vi "Three_Tote_works_3_21.vi"(11 "3_Tote_Enable":bool=TRUE) -> ()   [LabVIEW 2014]
uses:
  General_VI/Global Var.vi
panel:
  in  "Time _To_Drive_1_Tote":i32=8000
  in  "Extend_Flipper_Time":i32=500
  in  "Open_Infeed_time":i32=800
  # "Static Tunning Values"
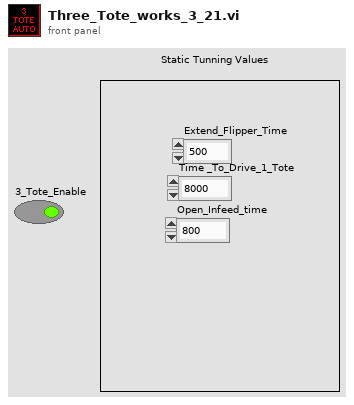
[diagram p1: front panel]
types:
  T1 = cluster{"Open_Infeed_time":i32, "Extend_Flipper_Time":i32, "Time _To_Drive_1_Tote":i32}
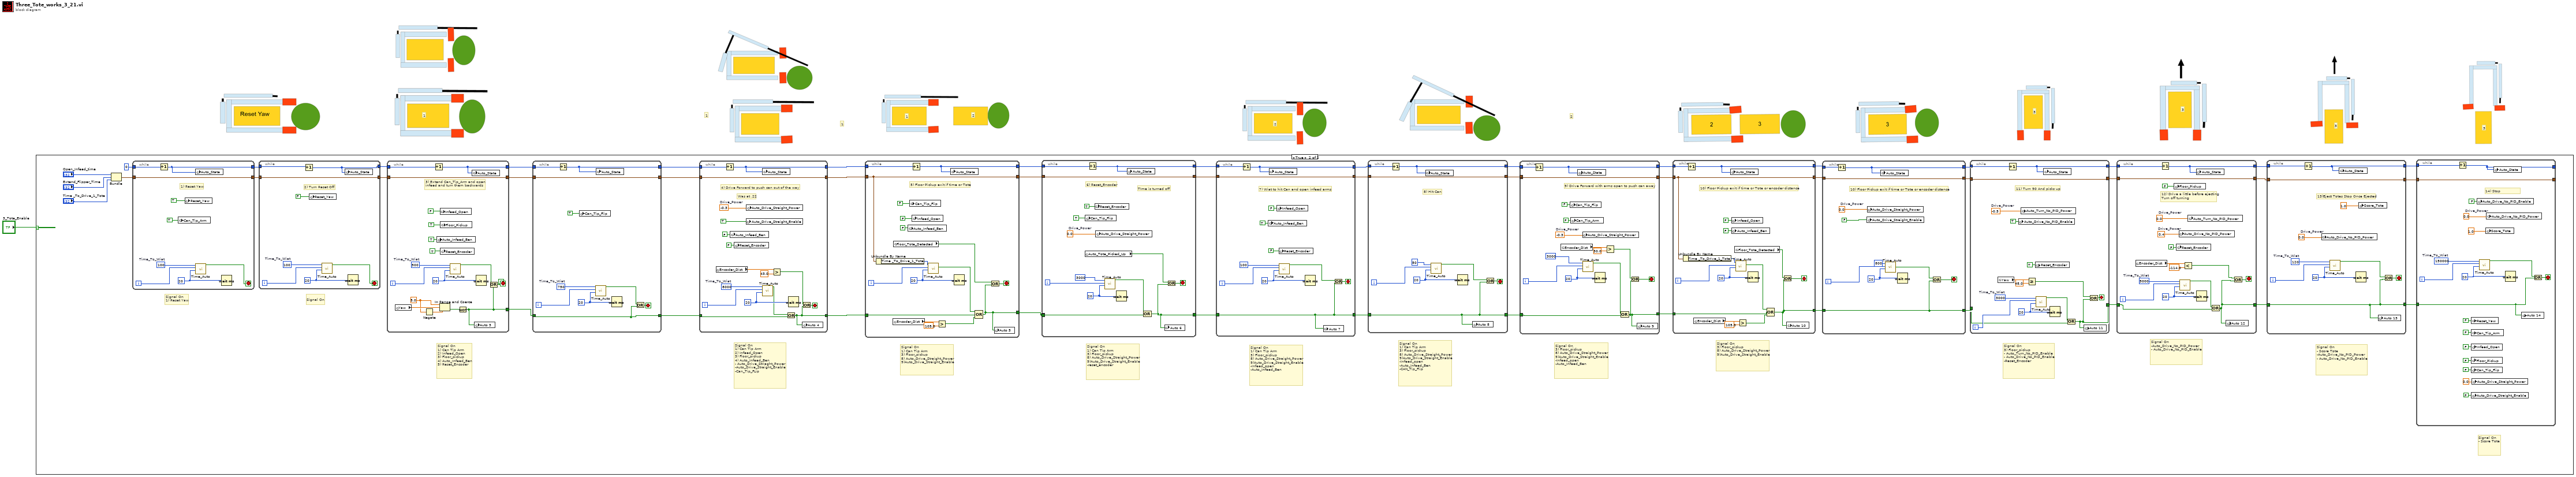
[diagram p0: block diagram]
diagram:
  # "3"
  # "3"
  # "3"
  # "3"
  # "2"
  # "2"
  # "2"
  # "1"
  # "1"
  # "1"
  # "1"
  n1 = case shown="True" "3_Tote_Enable" {
    frame False {
    }
    frame True {
      # "Signal On\n1) Can Tip Arm\n2) Infeed_Open\n3) Floor_pickup\n4) Auto_Infeed_Ben\n- Auto_Drive_Striaght_Power\n-Auto_Drive_Straight_Enable\n-Can_Tip_FLip"
      # "Signal On\n- Score Tote"
      # "Signal On\n- Score Tote\n-Auto_Drive_No_PID_Power\n- Auto_Drive_No_PID_Enable"
      # "Signal On\n-Auto_Drive_No_PID_Power\n- Auto_Drive_No_PID_Enable"
      # "Signal On\n3) Floor_pickup\n- Auto_Turn_No_PID_Enable\n- Auto_Drive_No_PID_Enable\n-Reset_Encoder"
      # "Signal On\n3) Floor_pickup\n8) Auto_Drive_Straight_Power\n9)Auto_Drive_Straight_Enable"
      # "Signal On\n3) Floor_pickup\n8) Auto_Drive_Straight_Power\n9)Auto_Drive_Straight_Enable\n-Infeed_open\n-Auto_Infeed_Ben"
      # "Signal On\n1) Can Tip Arm\n3) Floor_pickup\n8) Auto_Drive_Straight_Power\n9)Auto_Drive_Straight_Enable\n-Infeed_open\n-Auto_Infeed_Ben\n-CAN_Tip_Flip"
      # "Signal On\n1) Can Tip Arm\n3) Floor_pickup\n8) Auto_Drive_Straight_Power\n9)Auto_Drive_Straight_Enable\n-Infeed_open\n-Auto_Infeed_Ben"
      # "Signal On\n1) Can Tip Arm\n3) Floor_pickup\n8) Auto_Drive_Straight_Power\n9)Auto_Drive_Straight_Enable\n-reset_encoder"
      # "Signal On\n1) Can Tip Arm\n3) Floor_pickup\n8) Auto_Drive_Straight_Power\n9)Auto_Drive_Straight_Enable"
      # "Signal On\n1) Can Tip Arm\n2) Infeed_Open\n3) Floor_pickup\n4) Auto_Infeed_Ben\n5) Reset_Encoder"
      # "Signal On"
      # "Signal On\n1) Reset Yaw"
      n2 = Bundle("Open_Infeed_time"="Open_Infeed_time", "Extend_Flipper_Time"="Extend_Flipper_Time", "Time _To_Drive_1_Tote"="Time _To_Drive_1_Tote") -> (w39:T1)  [unwired: 1 in]
      n3 = while {
        tunnel: 0 -> [w262]
        tunnel: [w261] -> w48
        tunnel: w39 -> [w263]
        tunnel: [w263] -> w38
        i -> [w266]
        stop <- w268 stop-if-true
        w267 = u32 20 ("milliseconds to wait")
        w265 = 100  # Time_To_Wiat
        # "1) Reset Yaw"
        n4 = Increment(x=w262) -> (x+1=w261:i32)
        n5 = global write "Global Var.vi" "Can_Tip_Arm"(TRUE) -> ()
        n6 = global write "Global Var.vi" "Reset_Yaw"(TRUE) -> ()
        n7 = global write "Global Var.vi" "Auto_State"(w261) -> ()
        n8 = call "Time_Auto.vi"("Sample_Time"=w267, "Counter"=w266, "Time_to_wait"=w265) -> ("Boolean"=w268:bool)  [unwired: 8 in]
        n9 = Wait (ms)(milliseconds to wait=w267) -> ()  [unwired: 1 out]
      }
      n10 = while {
        tunnel: w48 -> [w253]
        tunnel: [w252] -> w47
        tunnel: w38 -> [w254]
        tunnel: [w254] -> w37
        i -> [w257]
        stop <- w259 stop-if-true
        w258 = u32 20 ("milliseconds to wait")
        w256 = 100  # Time_To_Wiat
        # "2) Turn Reset Off"
        n11 = Increment(x=w253) -> (x+1=w252:i32)
        n12 = global write "Global Var.vi" "Reset_Yaw"(FALSE) -> ()
        n13 = call "Time_Auto.vi"("Sample_Time"=w258, "Counter"=w257, "Time_to_wait"=w256) -> ("Boolean"=w259:bool)  [unwired: 8 in]
        n14 = global write "Global Var.vi" "Auto_State"(w252) -> ()
        n15 = Wait (ms)(milliseconds to wait=w258) -> ()  [unwired: 1 out]
      }
      n16 = while {
        tunnel: w47 -> [w247]
        tunnel: [w246] -> w11
        tunnel: w37 -> [w248]
        tunnel: [w248] -> w12
        tunnel: [w235] -> w14
        i -> [w250]
        stop <- w237 stop-if-true
        w241 = 5.0 ("upper limit")
        w251 = u32 20 ("milliseconds to wait")
        w249 = 500  # Time_To_Wiat
        # "3) Extend Can_Tip_Arm and open \ninfeed and turn them backwards"
        n17 = global read "Global Var.vi" "Yaw"() -> (w243:dbl)
        n18 = Negate(x=w241) -> (-x=w242:dbl)
        n19 = Increment(x=w247) -> (x+1=w246:i32)
        n20 = global write "Global Var.vi" "Auto_Infeed_Ben"(TRUE) -> ()
        n21 = In Range and Coerce(upper limit=w241, x=w243, lower limit=w242) -> (In Range?=w240:bool)  [unwired: 1 out]
        n22 = global write "Global Var.vi" "Infeed_Open"(FALSE) -> ()
        n23 = global write "Global Var.vi" "Floor_Pickup"(TRUE) -> ()
        n24 = global write "Global Var.vi" "Reset_Encoder"(TRUE) -> ()
        n25 = call "Time_Auto.vi"("Sample_Time"=w251, "Counter"=w250, "Time_to_wait"=w249) -> ("Boolean"=w236:bool)  [unwired: 8 in]
        n26 = Not(x=w240) -> (.not. x?=w235:bool)
        n27 = global write "Global Var.vi" "Auto_State"(w246) -> ()
        n28 = global write "Global Var.vi" "Auto 3"(w235) -> ()
        n29 = Wait (ms)(milliseconds to wait=w251) -> ()  [unwired: 1 out]
        n30 = Or(x=w236, y=w235) -> (x .or. y?=w237:bool)
      }
      n31 = while {
        tunnel: w11 -> [w66]
        tunnel: [w65] -> w10
        tunnel: w12 -> [w67]
        tunnel: [w67] -> w9
        tunnel: w14 -> [w61]
        tunnel: [w61] -> w13
        i -> [w69]
        stop <- w64 stop-if-true
        w70 = u32 20 ("milliseconds to wait")
        w68 = 750  # Time_To_Wiat
        n32 = Increment(x=w66) -> (x+1=w65:i32)
        n33 = global write "Global Var.vi" "Can_Tip_Flip"(TRUE) -> ()
        n34 = call "Time_Auto.vi"("Sample_Time"=w70, "Counter"=w69, "Time_to_wait"=w68) -> ("Boolean"=w62:bool)  [unwired: 8 in]
        n35 = global write "Global Var.vi" "Auto_State"(w65) -> ()
        n36 = Wait (ms)(milliseconds to wait=w70) -> ()  [unwired: 1 out]
        n37 = Or(x=w62, y=w61) -> (x .or. y?=w64:bool)
      }
      n38 = while {
        tunnel: w10 -> [w230]
        tunnel: [w229] -> w33
        tunnel: w9 -> [w231]
        tunnel: [w231] -> w32
        tunnel: w13 -> [w222]
        tunnel: [w219] -> w31
        i -> [w233]
        stop <- w221 stop-if-true
        w228 = -0.3  # Drive_Power
        w234 = u32 20 ("milliseconds to wait")
        w232 = 8000  # Time_To_Wiat
        # "Was at .22"
        # "4) Drive Forward to push can out of the way"
        n39 = global read "Global Var.vi" "Encoder_Dist"() -> (w225:dbl)
        n40 = Increment(x=w230) -> (x+1=w229:i32)
        n41 = global write "Global Var.vi" "Auto_Infeed_Ben"(FALSE) -> ()
        n42 = global write "Global Var.vi" "Reset_Encoder"(FALSE ("Reset_Encoder")) -> ()
        n43 = global write "Global Var.vi" "Auto_Drive_Straight_Enable"(TRUE) -> ()
        n44 = global write "Global Var.vi" "Auto_Drive_Straight_Power"(w228) -> ()
        n45 = call "Time_Auto.vi"("Sample_Time"=w234, "Counter"=w233, "Time_to_wait"=w232) -> ("Boolean"=w223:bool)  [unwired: 8 in]
        n46 = global write "Global Var.vi" "Auto_State"(w229) -> ()
        n47 = Greater?(x=w225, y=43.0) -> (0:w220:bool)
        n48 = Or(x=w223, y=w222) -> (x .or. y?=w219:bool)
        n49 = Wait (ms)(milliseconds to wait=w234) -> ()  [unwired: 1 out]
        n50 = Or(x=w220, y=w219) -> (x .or. y?=w221:bool)
        n51 = global write "Global Var.vi" "Auto 4"(w219) -> ()
      }
      n52 = while {
        tunnel: w33 -> [w215]
        tunnel: [w214] -> w30
        tunnel: w32 -> [w213]
        tunnel: [w213] -> w29
        tunnel: w31 -> [w211]
        tunnel: [w201] -> w2
        i -> [w216]
        stop <- w207 stop-if-true
        w217 = u32 20 ("milliseconds to wait")
        # "5) Floor Pickup exit if time or Tote"
        n53 = Unbundle By Name(w213) -> ("Time _To_Drive_1_Tote"=w212:i32)
        n54 = global read "Global Var.vi" "Encoder_Dist"() -> (w205:dbl)
        n55 = global read "Global Var.vi" "Floor_Tote_Detected"() -> (w206:bool)
        n56 = global write "Global Var.vi" "Auto_Infeed_Ben"(FALSE) -> ()
        n57 = global write "Global Var.vi" "Can_Tip_Flip"(FALSE) -> ()
        n58 = Increment(x=w215) -> (x+1=w214:i32)
        n59 = global write "Global Var.vi" "Infeed_Open"(FALSE) -> ()
        n60 = call "Time_Auto.vi"("Sample_Time"=w217, "Counter"=w216, "Time_to_wait"=w212) -> ("Boolean"=w210:bool)  [unwired: 8 in]
        n61 = Greater?(x=w205, y=105.0) -> (0:w204:bool)
        n62 = global write "Global Var.vi" "Auto_State"(w214) -> ()
        n63 = Wait (ms)(milliseconds to wait=w217) -> ()  [unwired: 1 out]
        n64 = Compound Arithmetic op=OR(w210, w211, w204) -> (w201:bool)
        n65 = Or(x=w206, y=w201) -> (x .or. y?=w207:bool)
        n66 = global write "Global Var.vi" "Auto 5"(w201) -> ()
      }
      n67 = while {
        tunnel: w30 -> [w98]
        tunnel: [w97] -> w15
        tunnel: w29 -> [w96]
        tunnel: [w96] -> w22
        tunnel: w2 -> [_]
        tunnel: [w88] -> w28
        tunnel: w2 -> [w89]
        i -> [w99]
        stop <- w95 stop-if-true
        w91 = 0.0  # Drive_Power
        w100 = u32 20 ("milliseconds to wait")
        # "TIme is turned off"
        # "6) Reset_Encoder"
        n68 = global read "Global Var.vi" "Auto_Tote_Picked_Up"() -> (w92:bool)
        n69 = global write "Global Var.vi" "Can_Tip_Flip"(TRUE) -> ()
        n70 = Increment(x=w98) -> (x+1=w97:i32)
        n71 = global write "Global Var.vi" "Reset_Encoder"(TRUE) -> ()
        n72 = global write "Global Var.vi" "Auto_Drive_Straight_Power"(w91) -> ()
        n73 = call "Time_Auto.vi"("Sample_Time"=w100, "Counter"=w99, "Time_to_wait"=3000) -> ("Boolean"=w90:bool)  [unwired: 8 in]
        n74 = Wait (ms)(milliseconds to wait=w100) -> ()  [unwired: 1 out]
        n75 = global write "Global Var.vi" "Auto_State"(w97) -> ()
        n76 = Compound Arithmetic op=OR(w90, w89) -> (w88:bool)
        n77 = global write "Global Var.vi" "Auto 6"(w88) -> ()
        n78 = Or(x=w92, y=w88) -> (x .or. y?=w95:bool)
      }
      n79 = while {
        tunnel: [w198] -> w46
        tunnel: w28 -> [w189]
        tunnel: [w189] -> w27
        tunnel: w22 -> [w191]
        tunnel: [w191] -> w21
        tunnel: w15 -> [w190]
        i -> [w199]
        stop <- w196 stop-if-true
        w200 = u32 20 ("milliseconds to wait")
        # "7) Wiat to hit Can and open infeed arms"
        n80 = Increment(x=w190) -> (x+1=w198:i32)
        n81 = global write "Global Var.vi" "Auto_Infeed_Ben"(TRUE) -> ()
        n82 = global write "Global Var.vi" "Auto_State"(w198) -> ()
        n83 = global write "Global Var.vi" "Infeed_Open"(FALSE ("Infeed_Open")) -> ()
        n84 = global write "Global Var.vi" "Reset_Encoder"(FALSE) -> ()
        n85 = call "Time_Auto.vi"("Sample_Time"=w200, "Counter"=w199, "Time_to_wait"=100) -> ("Boolean"=w195:bool)  [unwired: 8 in]
        n86 = Wait (ms)(milliseconds to wait=w200) -> ()  [unwired: 1 out]
        n87 = global write "Global Var.vi" "Auto 7"(w189) -> ()
        n88 = Or(x=w195, y=w189) -> (x .or. y?=w196:bool)
      }
      n89 = while {
        tunnel: w46 -> [w186]
        tunnel: [w185] -> w26
        tunnel: w27 -> [w180]
        tunnel: [w180] -> w24
        tunnel: w21 -> [w182]
        tunnel: [w182] -> w20
        i -> [w187]
        stop <- w184 stop-if-true
        w188 = u32 20 ("milliseconds to wait")
        # "8) HIt Can"
        n90 = Increment(x=w186) -> (x+1=w185:i32)
        n91 = global write "Global Var.vi" "Auto_State"(w185) -> ()
        n92 = call "Time_Auto.vi"("Sample_Time"=w188, "Counter"=w187, "Time_to_wait"=50) -> ("Boolean"=w183:bool)  [unwired: 8 in]
        n93 = Wait (ms)(milliseconds to wait=w188) -> ()  [unwired: 1 out]
        n94 = global write "Global Var.vi" "Auto 8"(w180) -> ()
        n95 = Or(x=w183, y=w180) -> (x .or. y?=w184:bool)
      }
      n96 = while {
        tunnel: [w83] -> w25
        tunnel: w26 -> [w82]
        tunnel: w24 -> [w79]
        tunnel: [w72] -> w23
        tunnel: [w74] -> _
        tunnel: w20 -> [w74]
        tunnel: [w74] -> w19
        i -> [w85]
        stop <- w84 stop-if-true
        w71 = -0.3  # Drive_Power
        w86 = u32 20 ("milliseconds to wait")
        # "9) Drive Forward with arms open to push can away"
        n97 = Increment(x=w82) -> (x+1=w83:i32)
        n98 = global read "Global Var.vi" "Encoder_Dist"() -> (w78:dbl)
        n99 = global write "Global Var.vi" "Can_Tip_Flip"(FALSE ("Infeed_Open")) -> ()
        n100 = global write "Global Var.vi" "Can_Tip_Arm"(FALSE ("Infeed_Open")) -> ()
        n101 = global write "Global Var.vi" "Auto_State"(w83) -> ()
        n102 = global write "Global Var.vi" "Auto_Drive_Straight_Power"(w71) -> ()
        n103 = call "Time_Auto.vi"("Sample_Time"=w86, "Counter"=w85, "Time_to_wait"=3000) -> ("Boolean"=w81:bool)  [unwired: 8 in]
        n104 = Wait (ms)(milliseconds to wait=w86) -> ()  [unwired: 1 out]
        n105 = Greater?(x=w78, y=30.0) -> (0:w76:bool)
        n106 = Compound Arithmetic op=OR(w81, w79) -> (w72:bool)
        n107 = Or(x=w76, y=w72) -> (x .or. y?=w84:bool)
        n108 = global write "Global Var.vi" "Auto 9"(w72) -> ()
      }
      n109 = while {
        tunnel: [w175] -> w8
        tunnel: [w164] -> w5
        tunnel: w25 -> [w172]
        tunnel: w23 -> [w169]
        tunnel: w19 -> [w167]
        tunnel: [w167] -> w3
        i -> [w178]
        stop <- w177 stop-if-true
        w179 = u32 20 ("milliseconds to wait")
        # "10) Floor Pickup exit if time or Tote or encoder distance"
        n110 = Unbundle By Name(w167) -> ("Time _To_Drive_1_Tote"=w174:i32)
        n111 = Increment(x=w172) -> (x+1=w175:i32)
        n112 = global read "Global Var.vi" "Encoder_Dist"() -> (w170:dbl)
        n113 = global write "Global Var.vi" "Auto_State"(w175) -> ()
        n114 = global write "Global Var.vi" "Infeed_Open"(FALSE ("Infeed_Open")) -> ()
        n115 = global write "Global Var.vi" "Auto_Infeed_Ben"(FALSE) -> ()
        n116 = global read "Global Var.vi" "Floor_Tote_Detected"() -> (w176:bool)
        n117 = call "Time_Auto.vi"("Sample_Time"=w179, "Counter"=w178, "Time_to_wait"=w174) -> ("Boolean"=w173:bool)  [unwired: 8 in]
        n118 = Greater?(x=w170, y=105.0) -> (0:w168:bool)
        n119 = Wait (ms)(milliseconds to wait=w179) -> ()  [unwired: 1 out]
        n120 = Compound Arithmetic op=OR(w173, w169, w168) -> (w164:bool)
        n121 = Or(x=w176, y=w164) -> (x .or. y?=w177:bool)
        n122 = global write "Global Var.vi" "Auto 10"(w164) -> ()
      }
      n123 = while {
        tunnel: [w58] -> w7
        tunnel: w8 -> [w57]
        tunnel: w3 -> [w56]
        tunnel: [w56] -> w6
        tunnel: w5 -> [w53]
        tunnel: [w53] -> w4
        i -> [w59]
        stop <- w55 stop-if-true
        w51 = 0.0  # Drive_Power
        w60 = u32 20 ("milliseconds to wait")
        # "10) Floor Pickup exit if time or Tote or encoder distance"
        n124 = Increment(x=w57) -> (x+1=w58:i32)
        n125 = global write "Global Var.vi" "Auto_Drive_Straight_Enable"(FALSE) -> ()
        n126 = global write "Global Var.vi" "Auto_Drive_Straight_Power"(w51) -> ()
        n127 = global write "Global Var.vi" "Auto_State"(w58) -> ()
        n128 = call "Time_Auto.vi"("Sample_Time"=w60, "Counter"=w59, "Time_to_wait"=800) -> ("Boolean"=w54:bool)  [unwired: 8 in]
        n129 = Wait (ms)(milliseconds to wait=w60) -> ()  [unwired: 1 out]
        n130 = Or(x=w54, y=w53) -> (x .or. y?=w55:bool)
      }
      n131 = while {
        tunnel: w7 -> [w161]
        tunnel: [w160] -> w45
        tunnel: w4 -> [w152]
        tunnel: [w148] -> w36
        tunnel: w6 -> [w157]
        tunnel: [w157] -> w18
        i -> [w153]
        stop <- w150 stop-if-true
        w155 = u32 20 ("milliseconds to wait")
        w154 = 3000  # Time_To_Wiat
        w159 = -0.5  # Drive_Power
        # "11) Turn 90 And picks up"
        n132 = global read "Global Var.vi" "Yaw"() -> (w163:dbl)
        n133 = Increment(x=w161) -> (x+1=w160:i32)
        n134 = global write "Global Var.vi" "Auto_Drive_No_PID_Enable"(TRUE ("Auto_Drive_No_PID_Enable")) -> ()
        n135 = global write "Global Var.vi" "Auto_Turn_No_PID_Power"(w159) -> ()
        n136 = Greater Or Equal?(x=w163, y=48.0) -> (x >= y?=w149:bool)
        n137 = global write "Global Var.vi" "Reset_Encoder"(TRUE ("Reset_Encoder")) -> ()
        n138 = call "Time_Auto.vi"("Sample_Time"=w155, "Counter"=w153, "Time_to_wait"=w154) -> ("Boolean"=w151:bool)  [unwired: 8 in]
        n139 = global write "Global Var.vi" "Auto_State"(w160) -> ()
        n140 = Wait (ms)(milliseconds to wait=w155) -> ()  [unwired: 1 out]
        n141 = Compound Arithmetic op=OR(w151, w152) -> (w148:bool)
        n142 = global write "Global Var.vi" "Auto 11"(w148) -> ()
        n143 = Or(x=w149, y=w148) -> (x .or. y?=w150:bool)
      }
      n144 = while {
        tunnel: w45 -> [w143]
        tunnel: [w142] -> w44
        tunnel: w36 -> [w137]
        tunnel: [w131] -> w35
        tunnel: w18 -> [w140]
        tunnel: [w140] -> w17
        i -> [w146]
        stop <- w133 stop-if-true
        w141 = 0.0  # Drive_Power
        w144 = 0.4  # Drive_Power
        w147 = u32 20 ("milliseconds to wait")
        w145 = 5000  # Time_To_Wiat
        # "12) Drive a little before ejecting\nTurn off turning"
        n145 = global read "Global Var.vi" "Encoder_Dist"() -> (w135:dbl)
        n146 = Increment(x=w143) -> (x+1=w142:i32)
        n147 = global write "Global Var.vi" "Floor_Pickup"(FALSE) -> ()
        n148 = global write "Global Var.vi" "Reset_Encoder"(FALSE ("Reset_Encoder")) -> ()
        n149 = global write "Global Var.vi" "Auto_Drive_No_PID_Power"(w144) -> ()
        n150 = call "Time_Auto.vi"("Sample_Time"=w147, "Counter"=w146, "Time_to_wait"=w145) -> ("Boolean"=w138:bool)  [unwired: 8 in]
        n151 = Less?(x=w135, y=-114.0) -> (x < y?=w132:bool)
        n152 = global write "Global Var.vi" "Auto_Turn_No_PID_Power"(w141) -> ()
        n153 = global write "Global Var.vi" "Auto_State"(w142) -> ()
        n154 = Wait (ms)(milliseconds to wait=w147) -> ()  [unwired: 1 out]
        n155 = Compound Arithmetic op=OR(w138, w137) -> (w131:bool)
        n156 = global write "Global Var.vi" "Auto 12"(w131) -> ()
        n157 = Or(x=w132, y=w131) -> (x .or. y?=w133:bool)
      }
      n158 = while {
        tunnel: w44 -> [w126]
        tunnel: [w125] -> w43
        tunnel: w35 -> [w120]
        tunnel: [w120] -> w34
        tunnel: w17 -> [w123]
        tunnel: [w123] -> w16
        i -> [w129]
        stop <- w122 stop-if-true
        w124 = 0.0  # Drive_Power
        w130 = u32 20 ("milliseconds to wait")
        w128 = 120  # Time_To_Wiat
        # "13)Eject Totes Stop Once Ejected"
        n159 = Increment(x=w126) -> (x+1=w125:i32)
        n160 = global write "Global Var.vi" "Auto_Drive_No_PID_Power"(w124) -> ()
        n161 = call "Time_Auto.vi"("Sample_Time"=w130, "Counter"=w129, "Time_to_wait"=w128) -> ("Boolean"=w121:bool)  [unwired: 8 in]
        n162 = global write "Global Var.vi" "Auto_State"(w125) -> ()
        n163 = Wait (ms)(milliseconds to wait=w130) -> ()  [unwired: 1 out]
        n164 = global write "Global Var.vi" "Score_Tote"(1.0) -> ()
        n165 = global write "Global Var.vi" "Auto 13"(w120) -> ()
        n166 = Or(x=w121, y=w120) -> (x .or. y?=w122:bool)
      }
      n167 = while {
        tunnel: w43 -> [w115]
        tunnel: [w114] -> _
        tunnel: w34 -> [w101]
        tunnel: w16 -> [w104]
        tunnel: [w104] -> _
        i -> [w118]
        stop <- w103 stop-if-true
        w112 = 0.0  # Drive_Power
        w119 = u32 20 ("milliseconds to wait")
        w117 = 150000  # Time_To_Wiat
        # "14) Stop"
        n168 = Increment(x=w115) -> (x+1=w114:i32)
        n169 = global write "Global Var.vi" "Reset_Yaw"(FALSE ("Reset_Yaw")) -> ()
        n170 = global write "Global Var.vi" "Can_Tip_Arm"(FALSE ("Can_Tip_Arm")) -> ()
        n171 = global write "Global Var.vi" "Infeed_Open"(FALSE ("Infeed_Open")) -> ()
        n172 = global write "Global Var.vi" "Floor_Pickup"(FALSE ("Floor_Pickup")) -> ()
        n173 = global write "Global Var.vi" "Can_Tip_Flip"(FALSE ("Can_Tip_Flip")) -> ()
        n174 = global write "Global Var.vi" "Auto_Drive_Straight_Enable"(FALSE ("Auto_Drive_Straight_Enable")) -> ()
        n175 = global write "Global Var.vi" "Auto_Drive_Straight_Power"(0.0 ("Auto_Drive_Straight_Power")) -> ()
        n176 = global write "Global Var.vi" "Auto_Drive_No_PID_Enable"(FALSE ("Auto_Drive_No_PID_Enable")) -> ()
        n177 = call "Time_Auto.vi"("Sample_Time"=w119, "Counter"=w118, "Time_to_wait"=w117) -> ("Boolean"=w102:bool)  [unwired: 8 in]
        n178 = global write "Global Var.vi" "Score_Tote"(1.0) -> ()
        n179 = global write "Global Var.vi" "Auto_Drive_No_PID_Power"(w112) -> ()
        n180 = global write "Global Var.vi" "Auto_State"(w114) -> ()
        n181 = Wait (ms)(milliseconds to wait=w119) -> ()  [unwired: 1 out]
        n182 = global write "Global Var.vi" "Auto 14"(w101) -> ()
        n183 = Or(x=w102, y=w101) -> (x .or. y?=w103:bool)
      }
    }
  }
